vi "LvMPDC_SUB_PropertyPanel.vi"(10 "MusicInfo":T1 {"time" format="%<%H:%M:%S%3u>t"}) -> ()   [LabVIEW 2012]
uses:
  LvMPDC_Typdef_MusicInfo.ctl
  <vilib>/Utility/miscctls.llb/LVPointTypeDef.ctl
panel:
  out "PropertyList":i32(listbox)
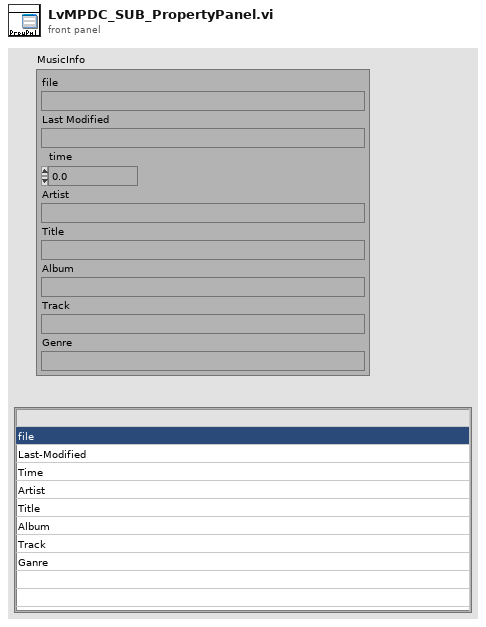
[diagram p1: front panel]
types:
  T1 = typedef "LvMPDC_Typdef_MusicInfo.ctl" = cluster{"file":string, "Last Modified":string, "time":dbl, "Artist":string, "Title":string, "Album":string, "Track":string, "Genre":string}
  T2 = typedef "LVPointTypeDef.ctl" = cluster{"Horizontal":i16, "Vertical":i16}
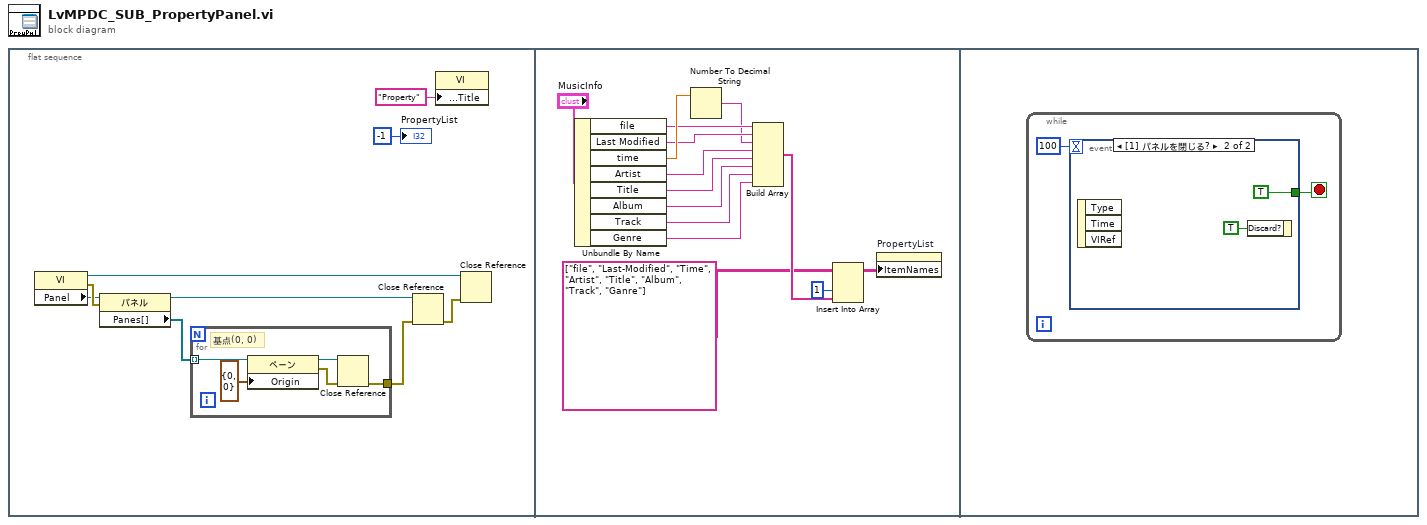
[diagram p0: block diagram]
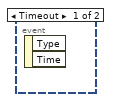
[diagram p2: hidden frame]
diagram:
  n1 = flat-sequence {
    frame #0 {
      n2 = property class="VI"() -> (reference out=w4:refnum<vi>, error out=w7:errorcluster, "Panel"=w1:refnum<vi>)  [unwired: 2 in]
      n3 = property on="プロパティノード" class="パネル"(reference=w1, error in=w7) -> (reference out=w3:refnum<vi>, "Panes[]"=w2:refnum<vi>[])  [unwired: 1 out]
      n4 = for {
        tunnel: w2 -> [w14] mode=indexing
        tunnel: [w11] -> w5
        # "基点(0, 0)"
        n5 = property on="プロパティノード" class="ペーン"(reference=w14, "Origin"=T2 {"Horizontal"=0, "Vertical"=0} ("原点")) -> (reference out=w13:refnum<vi>, error out=w12:errorcluster)  [unwired: 1 in]
        n6 = Close Reference(reference=w13, error in (no error)=w12) -> (error out=w11:errorcluster)
      }
      n7 = Close Reference(reference=w3, error in (no error)=w5) -> (error out=w6:errorcluster)
      n8 = property class="VI"("Front Panel.Title"="Property" ("フロントパネルウィンドウ:タイトル")) -> ()  [unwired: 2 in, 2 out]
      n9 = Close Reference(reference=w4, error in (no error)=w6) -> ()  [unwired: 1 out]
      "PropertyList" <- -1 ("PropertyList")
    }
    frame #1 {
      n10 = Unbundle By Name("MusicInfo") -> ("file"=w27:string, "Last Modified"=w26:string, "time"=w28:dbl, "Artist"=w25:string, "Title"=w24:string, "Album"=w23:string, "Track"=w22:string, "Genre"=w21:string)
      n11 = Number To Decimal String(number=w28) -> (decimal integer string=w20:string)  [unwired: 1 in]
      n12 = Build Array(w27, w26, w20, w25, w24, w23, w22, w21) -> (w17:string[])
      n13 = Insert Into Array(array=string[][] [["file"], ["Last-Modified"], ["Time"], ["Artist"], ["Title"], ["Album"], ["Track"], ["Ganre"]] ("項目名"), index (col)=1 ("無効な指標 （列）"), new element=w17) -> (w15:string[][])  [unwired: 1 in]
      n14 = property on="PropertyList" class="MCListbox （指定）"("ItemNames"=w15) -> ()  [unwired: 2 in, 2 out]
    }
    frame #2 {
      n15 = while {
        stop <- w29 stop-if-true
        n16 = event shown="[1] パネルを閉じる?" {
          selector: _ -> [_ _]
          dyn-events: _ -> [_ _]
          timeout: 100 -> [_ _]
          tunnel: [_ TRUE] -> w29
          event Timeout {
            n17 = event-data() -> ()  [unwired: 1 in, 2 out]
          }
          event Panel Close? {
            n18 = event-data() -> ()  [unwired: 1 in, 3 out]
            n19 = event-data("Discard?"=TRUE ("破棄?")) -> ()  [unwired: 1 in, 1 out]
          }
        }
      }
    }
  }
